vi "WriteKeyIfValueExists.vi"(7 "section":string, 8 "error in (no error)":errorcluster, 9 "value":string, 10 "key":string, 11 "refnum out":T1) -> (0 "error out":errorcluster, 2 "found?":bool, 3 "refnum out":T1)   [LabVIEW 2015]
doc: "Use this template to build a VI to use as a subVI."
uses:
  <vilib>/Utility/config.llb/Config Data RefNum.ctl
  <vilib>/Utility/config.llb/Write Key (String).vi
  <vilib>/Utility/config.llb/NI_LVConfig.lvlib
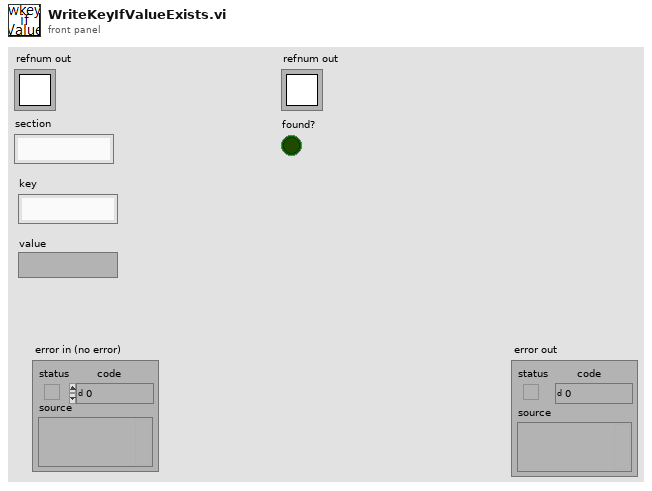
[diagram p1: front panel]
types:
  T1 = typedef "NI_LVConfig.lvlib/Config Data RefNum.ctl" = refnum<k1>
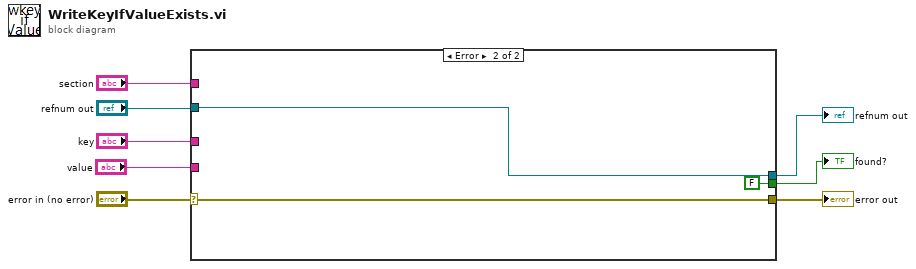
[diagram p0: block diagram]
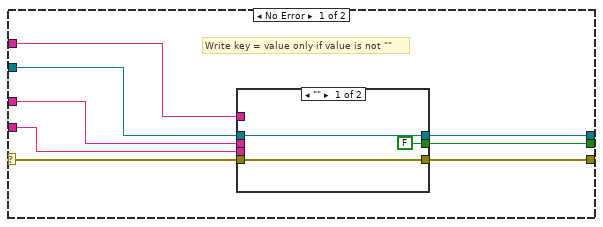
[diagram p2: hidden frame]
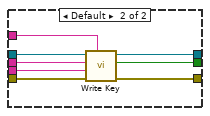
[diagram p3: hidden frame]
diagram:
  n1 = case shown="Error" "error in (no error)" {
    selector: "error in (no error)" -> [w15 w30]
    tunnel: [w14 w30] -> w7
    tunnel: "refnum out" -> [w16 w28]
    tunnel: "section" -> [w12 _]
    tunnel: "key" -> [w13 _]
    tunnel: "value" -> [w11 _]
    tunnel: [w10 w28] -> w1
    tunnel: [w9 FALSE ("found?")] -> w2
    frame No Error {
      # "Write key = value only if value is not \"\""
      n2 = case shown="\"\"" w11 {
        selector: w11 -> [_ w22]
        tunnel: w16 -> [w18 w27]
        tunnel: w15 -> [w19 w26]
        tunnel: [w19 w25] -> w14
        tunnel: w11 -> [_ _]
        tunnel: w13 -> [_ w24]
        tunnel: w12 -> [_ w23]
        tunnel: [w18 w21] -> w10
        tunnel: [FALSE ("found?") w20] -> w9
        frame "" {
        }
        frame Default {
          n3 = call-poly <vilib>:"Write Key.vi"("section"=w23, "error in (no error)"=w26, "value"=w22, "key"=w24, "refnum"=w27) -> ("error out"=w25:errorcluster, "found?"=w20:bool, "refnum out"=w21:T1)  [unwired: 4 in]
        }
      }
    }
    frame Error {
    }
  }
  "error out" <- w7
  "refnum out" <- w1
  "found?" <- w2
